vi "Get Scanner.vi"(8 "error in (no error)":errorcluster, 11 "Analog Output in":refnum<class "Analog Output.lvclass">) -> (0 "error out":errorcluster, 2 "Default Scanner out":refnum<class "Scanner.lvclass">)   [LabVIEW 2017, in "Analog Output.lvclass"]
doc: "(Dynamic) Returns the default Scanner object that scans over this Scannable. (Note that a Scannable may have multiple Scanners associated with it.) A Scanner is an analogue to an Iterator class in other languages."
uses:
  Analog Output.lvclass
  Scanners/Scanner/Scanner.lvclass
  Scanners/Analog Out Scan/Analog Out Scan.lvclass
  C:/LabVIEW-programs-dev/Scanners/Scanner/Scanner.lvclass
  Utility Classes/Scannable/Scannable.lvclass
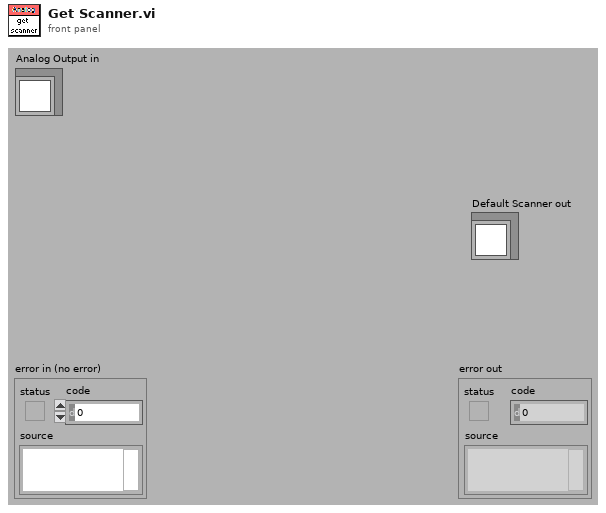
[diagram p1: front panel]
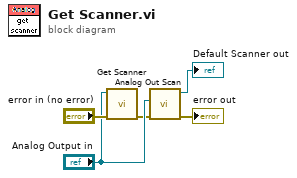
[diagram p0: block diagram]
diagram:
  n1 = call-parent "Get Scanner.vi"("error in (no error)"="error in (no error)", "Scannable in"="Analog Output in") -> ("error out"=w2:errorcluster)  [unwired: 8 in, 1 out]
  n2 = call "Analog Out Scan.vi"("error in (no error)"=w2, "Analog Output.lvclass"="Analog Output in") -> ("error out"=→"error out":errorcluster, "Analog Out Scan out"=→"Default Scanner out":refnum<class "Analog Out Scan.lvclass">)  [unwired: 8 in]
